vi "NEWEST PI_1.vi"(0 "CtrlIndex":i32, 1 "ControlArray":T1(array[cluster]), 5 "CommandCluster":T3, 6 "Run?":bool, 7 "Feedback":dbl[](array[numeric]), 9 "VandPLimits":dbl[](array[numeric]), 11 "Stability In":T2, 12 "Tolerances":dbl[](array[numeric]), 13 "Controller?":bool, 14 "Ave Feedback":dbl[](array[numeric])) -> (4 "PIdata":dbl[](array[numeric]), 8 "Output":dbl, 10 "Stable?":bool, 15 "Stability Out":T2)   [LabVIEW 2013]
uses:
  TypeDef/Command Cluster.ctl
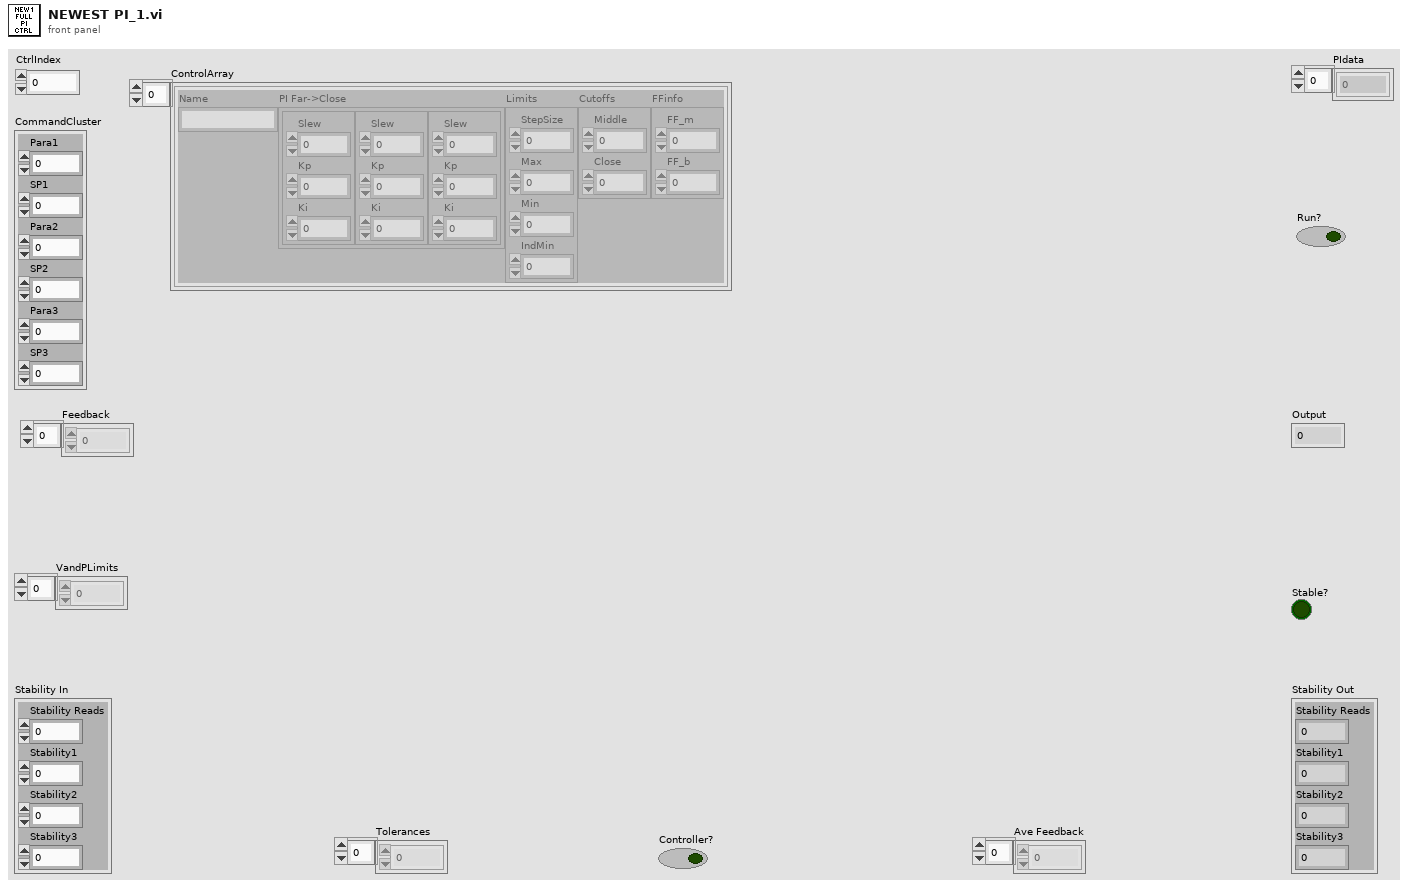
[diagram p1: front panel]
types:
  T1 = cluster{"Name":string, "PI Far->Close":cluster{"Slew":dbl, "Kp":dbl, "Ki":dbl}[], "Limits":cluster{"StepSize":dbl, "Max":dbl, "Min":dbl, "IndMin":dbl}, "Cutoffs":cluster{"Middle":dbl, "Close":dbl}, "FFinfo":cluster{"FF_m":dbl, "FF_b":dbl}}[]
  T2 = cluster{"Stability Reads":i32, "Stability1":i32, "Stability2":i32, "Stability3":i32}
  T3 = typedef "Command Cluster.ctl" = cluster{"Para1":i32, "SP1":dbl, "Para2":i32, "SP2":dbl, "Para3":i32, "SP3":dbl}
  T4 = cluster{"Name":string, "PI Far->Close":cluster{"Slew":dbl, "Kp":dbl, "Ki":dbl}[], "Limits":cluster{"StepSize":dbl, "Max":dbl, "Min":dbl, "IndMin":dbl}, "Cutoffs":cluster{"Middle":dbl, "Close":dbl}, "FFinfo":cluster{"FF_m":dbl, "FF_b":dbl}}
  T5 = cluster{"StepSize":dbl, "Max":dbl, "Min":dbl, "IndMin":dbl}
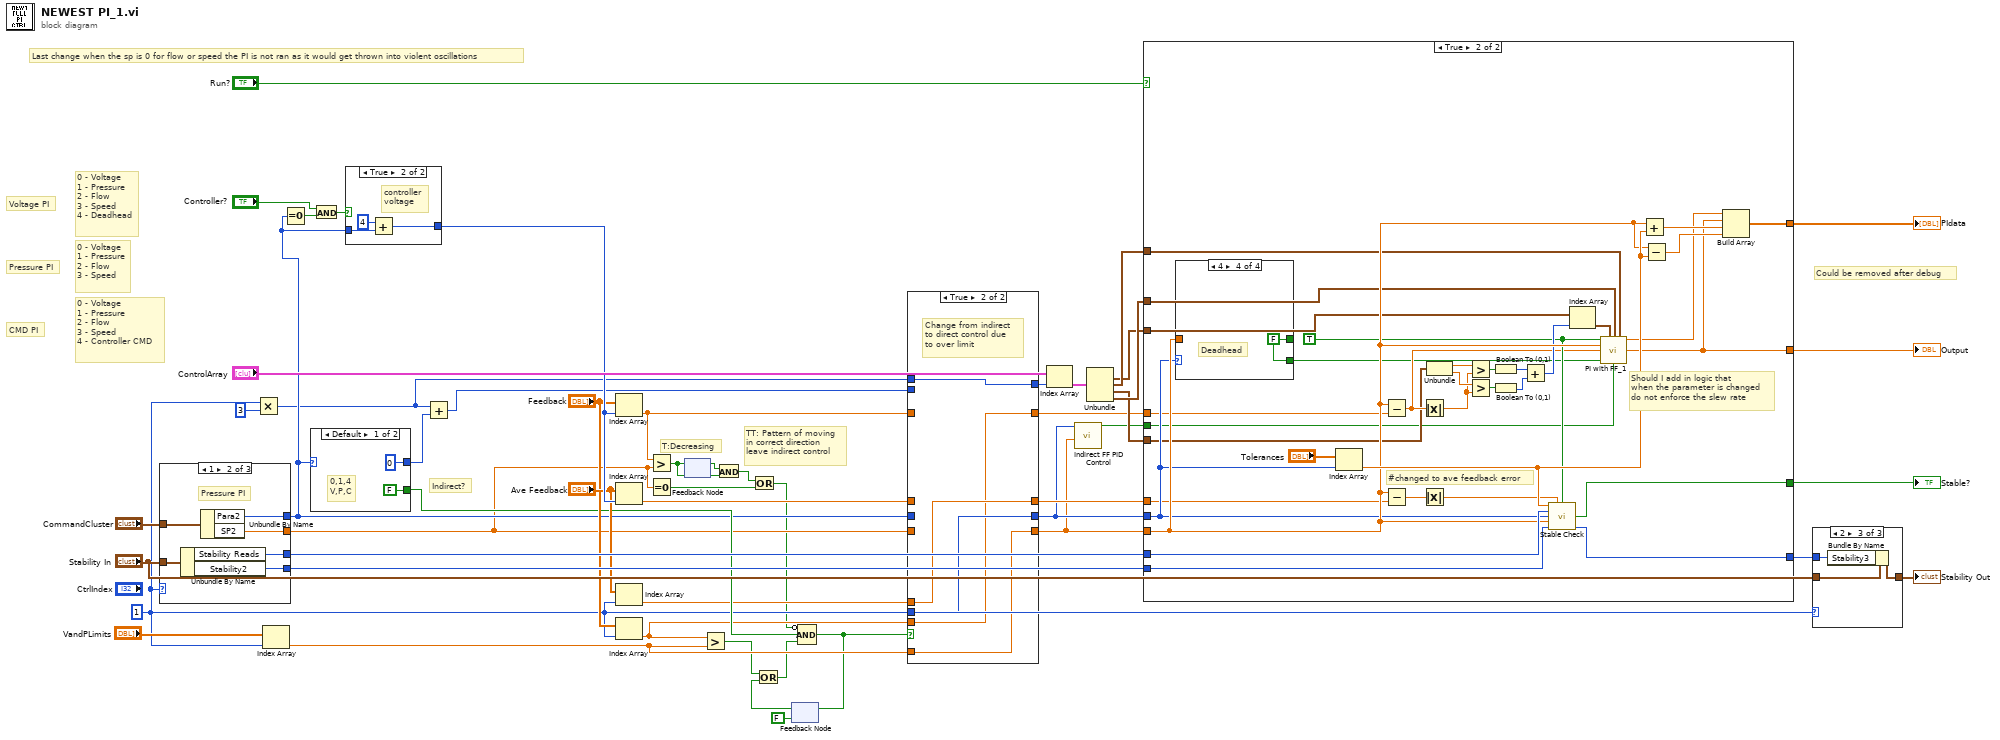
[diagram p0: block diagram]
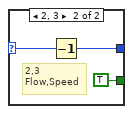
[diagram p4: hidden frame]
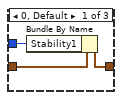
[diagram p5: hidden frame]
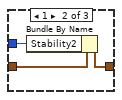
[diagram p6: hidden frame]
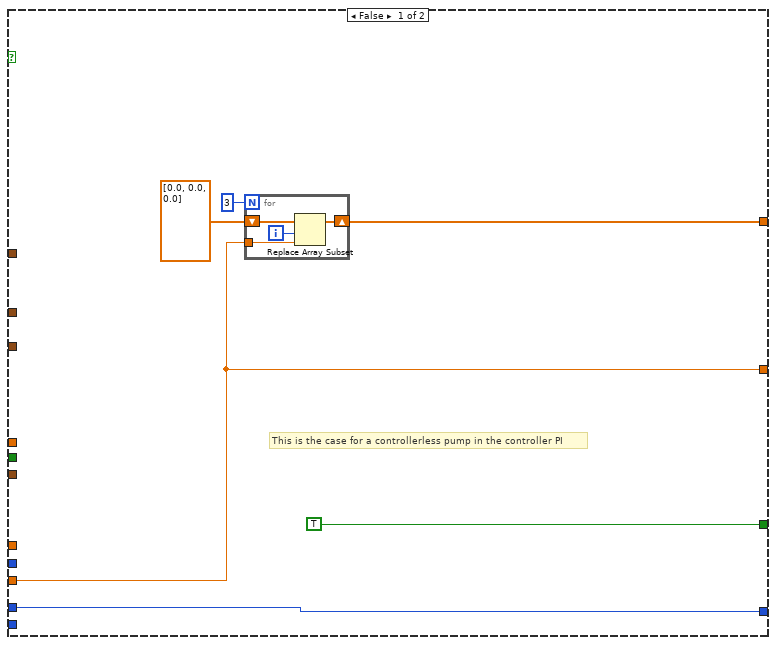
[diagram p7: hidden frame]
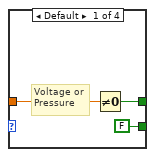
[diagram p8: hidden frame]
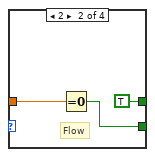
[diagram p9: hidden frame]
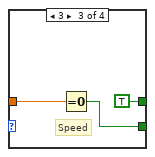
[diagram p10: hidden frame]
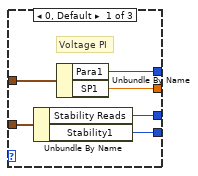
[diagram p11: hidden frame]
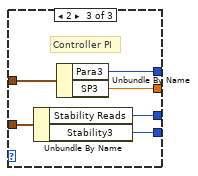
[diagram p12: hidden frame]
diagram:
  w21 = 1 ("CtrlIndex")
  # "TT: Pattern of moving\nin correct direction\nleave indirect control"
  # "T:Decreasing"
  # "Indirect?"
  # "Last change when the sp is 0 for flow or speed the PI is not ran as it would get thrown into violent oscillations"
  # "Could be removed after debug"
  # "CMD PI"
  # "Pressure PI"
  # "Voltage PI"
  # "0 - Voltage\n1 - Pressure\n2 - Flow\n3 - Speed\n4 - Controller CMD"
  # "0 - Voltage\n1 - Pressure\n2 - Flow\n3 - Speed"
  # "0 - Voltage\n1 - Pressure\n2 - Flow\n3 - Speed\n4 - Deadhead"
  n1 = case shown="1" w21 {
    tunnel: "Stability In" -> [w58 w64 w70]
    tunnel: [w56 w62 w68] -> w51
    tunnel: [w57 w63 w69] -> w50
    tunnel: "CommandCluster" -> [w55 w61 w67]
    tunnel: [w54 w60 w66] -> w23
    tunnel: [w53 w59 w65] -> w12
    frame 0, Default {
      # "Voltage PI"
      n2 = Unbundle By Name(w58) -> ("Stability Reads"=w56:i32, "Stability1"=w57:i32)
      n3 = Unbundle By Name(w55) -> ("Para1"=w54:i32, "SP1"=w53:dbl)
    }
    frame 1 {
      # "Pressure PI"
      n4 = Unbundle By Name(w64) -> ("Stability Reads"=w62:i32, "Stability2"=w63:i32)
      n5 = Unbundle By Name(w61) -> ("Para2"=w60:i32, "SP2"=w59:dbl)
    }
    frame 2 {
      # "Controller PI"
      n6 = Unbundle By Name(w70) -> ("Stability Reads"=w68:i32, "Stability3"=w69:i32)
      n7 = Unbundle By Name(w67) -> ("Para3"=w66:i32, "SP3"=w65:dbl)
    }
  }
  n8 = Multiply(x=w21, y=3) -> (x*y=w15:i32)
  n9 = Index Array(array="VandPLimits", index=w21) -> (element=w20:dbl)
  n10 = Equal To 0?(x=w23) -> (x = 0?=w33:bool)
  n11 = case shown="Default" w23 {
    selector: w23 -> [_ w75]
    tunnel: [0 w74] -> w35
    tunnel: [FALSE TRUE] -> w25
    frame Default {
      # "0,1,4\nV,P,C"
    }
    frame 2, 3 {
      # "2,3\nFlow,Speed"
      n12 = Decrement(x=w75) -> (x-1=w74:i32)
    }
  }
  n13 = And(x="Controller?", y=w33) -> (x .and. y?=w34:bool)
  n14 = case shown="True" w34 {
    tunnel: w23 -> [w76 w79]
    tunnel: [w76 w77] -> w30
    frame False {
      # "pump\nvoltage"
    }
    frame True {
      # "controller\nvoltage"
      n15 = Add(x=4, y=w79) -> (x+y=w77:i32)
    }
  }
  n16 = Add(x=w15, y=w35) -> (x+y=w14:i32)
  n17 = Index Array(array="Feedback", index=w30) -> (element=w17:dbl)
  n18 = Index Array(array="Ave Feedback", index=w30) -> (element=w24:dbl)
  n19 = Index Array(array="Ave Feedback", index=w21) -> (element=w18:dbl)
  n20 = Index Array(array="Feedback", index=w21) -> (element=w19:dbl)
  n21 = Greater?(x=w17, y=w12) -> (0:w27:bool)
  n22 = Equal To 0?(x=w12) -> (x = 0?=w11:bool)
  n23 = feedback #1(w27) -> (w26:bool)
  n24 = feedback-in #1(w27) -> ()
  n25 = Greater?(x=w19, y=w20) -> (0:w6:bool)
  n26 = And(x=w26, y=w27) -> (x .and. y?=w10:bool)
  n27 = Or(x=w10, y=w11) -> (x .or. y?=w9:bool)
  n28 = feedback #2(FALSE) -> (w7:bool)
  n29 = Or(x=w6, y=w7) -> (x .or. y?=w4:bool)
  n30 = Compound Arithmetic op=AND(invert w9, w25, w4) -> (w5:bool)
  n31 = feedback-in #2(w5) -> ()
  n32 = case shown="True" w5 {
    tunnel: w23 -> [w83 _]
    tunnel: w12 -> [w82 _]
    tunnel: [w83 w88] -> w2
    tunnel: [w82 w89] -> w1
    tunnel: w24 -> [w84 _]
    tunnel: [w84 w87] -> w22
    tunnel: w17 -> [w81 _]
    tunnel: [w81 w86] -> w16
    tunnel: w14 -> [w80 _]
    tunnel: [w80 w85] -> w13
    tunnel: w18 -> [_ w87]
    tunnel: w19 -> [_ w86]
    tunnel: w20 -> [_ w89]
    tunnel: w21 -> [_ w88]
    tunnel: w15 -> [_ w85]
    frame False {
      # "Leave controls as is"
    }
    frame True {
      # "Change from indirect\nto direct control due\nto over limit"
    }
  }
  n33 = Index Array(array="ControlArray", index=w13) -> (element=w40:T4)
  n34 = call "Indirect FF PID Control.vi"("Setpoint"=w1, "Parameter"=w2) -> ("Indirect FF"=w3:bool)  [unwired: 9 in]
  n35 = Unbundle(w40) -> ("PI Far->Close"=w36:cluster{"Slew":dbl, "Kp":dbl, "Ki":dbl}[], "Limits"=w38:T5, "Cutoffs"=w37:cluster{"Middle":dbl, "Close":dbl}, "FFinfo"=w39:cluster{"FF_m":dbl, "FF_b":dbl})  [unwired: 1 out]
  n36 = case shown="True" "Run?" {
    tunnel: w51 -> [w94 w124]
    tunnel: w50 -> [_ w123]
    tunnel: w2 -> [_ w106]
    tunnel: w1 -> [w93 w117]
    tunnel: [TRUE w120] -> w48
    tunnel: [w93 w104] -> w47
    tunnel: [w91 w132] -> w46
    tunnel: [w94 w125] -> w45
    tunnel: w38 -> [_ w109]
    tunnel: w39 -> [_ w108]
    tunnel: w37 -> [_ w105]
    tunnel: w36 -> [_ w107]
    tunnel: w22 -> [_ w102]
    tunnel: w16 -> [_ w101]
    tunnel: w3 -> [_ w100]
    frame False {
      # "This is the case for a controllerless pump in the controller PI"
      n37 = for {
        N: 3 -> [_]
        shift-right: [w98] -> w91
        shift-left: dbl[] [0.0, 0.0, 0.0] -> [w99]
        tunnel: w93 -> [w96]
        i -> [w97]
        n38 = Replace Array Subset(array=w99, new element=w96, index=w97) -> (w98:dbl[])
      }
    }
    frame True {
      w113 = TRUE
      # "#changed to ave feedback error"
      # "Should I add in logic that\nwhen the parameter is changed\ndo not enforce the slew rate"
      n39 = case shown="4" w106 {
        tunnel: [w134 TRUE TRUE w143] -> _
        tunnel: w117 -> [w135 w139 w142 _]
        tunnel: [FALSE w138 w141 w143] -> w111
        frame Default {
          # "Voltage or\nPressure"
          n40 = Not Equal To 0?(x=w135) -> (x != 0?=w134:bool)
        }
        frame 2 {
          # "Flow"
          n41 = Equal To 0?(x=w139) -> (x = 0?=w138:bool)
        }
        frame 3 {
          # "Speed"
          n42 = Equal To 0?(x=w142) -> (x = 0?=w141:bool)
        }
        frame 4 {
          w143 = FALSE
          # "Deadhead"
        }
      }
      n43 = Index Array(array="Tolerances", index=w106) -> (element=w119:dbl)
      n44 = Subtract(x=w117, y=w101) -> (x-y=w112:dbl)
      n45 = Subtract(x=w117, y=w102) -> (x-y=w122:dbl)
      n46 = Absolute Value(x=w112) -> (abs(x)=w121:dbl)
      n47 = Absolute Value(x=w122) -> (abs(x)=w118:dbl)
      n48 = Unbundle(w105) -> ("Middle"=w127:dbl, "Close"=w126:dbl)
      n49 = Greater?(x=w127, y=w121) -> (0:w131:bool)
      n50 = Greater?(x=w126, y=w121) -> (0:w130:bool)
      n51 = Boolean To (0,1)(Boolean=w131) -> (0, 1=w129:i16)
      n52 = Boolean To (0,1)(Boolean=w130) -> (0, 1=w128:i16)
      n53 = Add(x=w129, y=w128) -> (x+y=w114:i16)
      n54 = call "Stable Check.vi"("Tolerance"=w119, "AbsError"=w118, "PI Running?"=w113, "ReqReads"=w124, "Parameter"=w106, "Setpoint"=w117, "StabilityCount In"=w123) -> ("Stable?"=w120:bool, "StabilityCount Out"=w125:i32)  [unwired: 6 in, 1 out]
      n55 = Index Array(array=w107, index=w114) -> (element=w110:cluster{"Slew":dbl, "Kp":dbl, "Ki":dbl})
      n56 = call "PI with FF_1.vi"("Run PI?"=w113, "PIcluster"=w110, "FFcluster"=w108, "LimitCluster"=w109, "SP"=w117, "Error"=w112, "RevCtrlZero"=w111, "Indirect FF"=w100) -> ("PreSlew"=w103:dbl, "Output"=w104:dbl)  [unwired: 6 in]
      n57 = Add(x=w117, y=w119) -> (x+y=w116:dbl)
      n58 = Subtract(x=w117, y=w119) -> (x-y=w115:dbl)
      n59 = Build Array(w103, w104, w116, w115) -> (w132:dbl[])
    }
  }
  "Stable?" <- w48
  "Output" <- w47
  "PIdata" <- w46
  n60 = case shown="2" w21 {
    tunnel: "Stability In" -> [w145 w148 w151]
    tunnel: [w144 w147 w150] -> w49
    tunnel: w45 -> [w146 w149 w152]
    frame 0, Default {
      n61 = Bundle By Name(cluster=w145, "Stability1"=w146) -> (w144:T2)
    }
    frame 1 {
      n62 = Bundle By Name(cluster=w148, "Stability2"=w149) -> (w147:T2)
    }
    frame 2 {
      n63 = Bundle By Name(cluster=w151, "Stability3"=w152) -> (w150:T2)
    }
  }
  "Stability Out" <- w49
